vi "Insert_Event.vi"(0 "Alias Table":string[][](array[string])) -> (1 "Command":string, 2 "Cancelled":bool)   [LabVIEW 2011]
doc: "This modal VI functions as a popup window, allowing the user to select a new event to insert into the sequence."
panel:
  in  "Commands":i32(listbox)
  in  "Cancel":bool
  in  "OK":bool
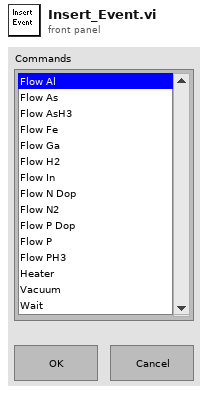
[diagram p1: front panel]
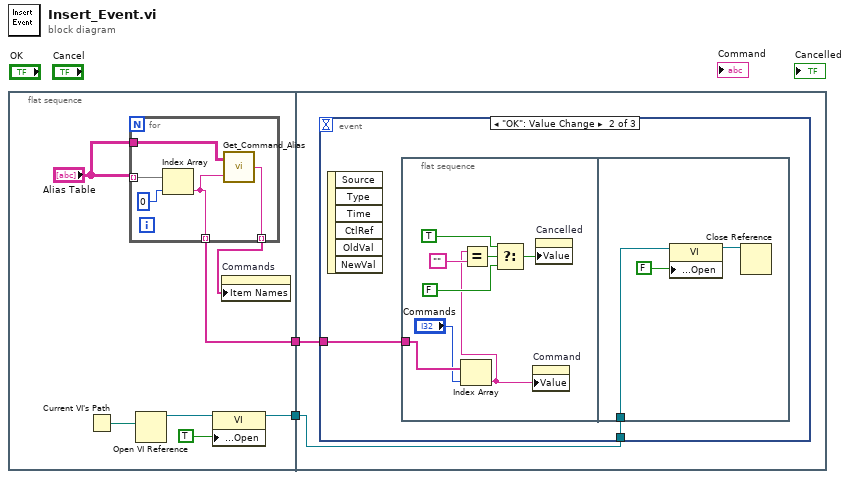
[diagram p0: block diagram]
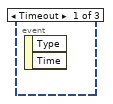
[diagram p2: hidden frame]
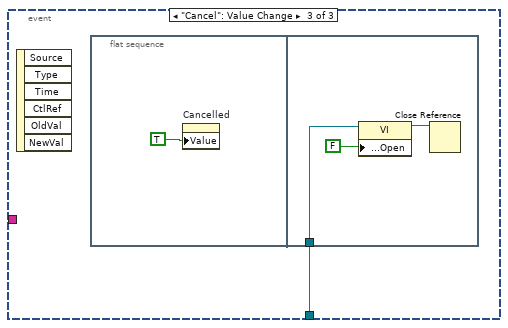
[diagram p3: hidden frame]
diagram:
  n1 = flat-sequence {
    tunnel: [w8] -> w2
    tunnel: [w4] -> w1
    tunnel: w2 -> [w16]
    tunnel: w1 -> [w15]
    frame #0 {
      n2 = Current VI's Path() -> (path=w6:path)
      n3 = for {
        tunnel: "Alias Table" -> [w13]
        tunnel: [w14] -> w5 mode=indexing
        tunnel: [w10] -> w4 mode=indexing
        tunnel: "Alias Table" -> [w12] mode=indexing
        n4 = Index Array(array=w12, index=0) -> (element=w10:string)
        n5 = call "Get_Command_Alias.vi"("Command"=w10, "Alias Table"=w13) -> ("Alias"=w14:string)
      }
      n6 = Open VI Reference(vi path=w6) -> (vi reference=w7:refnum<vi>)  [unwired: 1 in, 5 out]
      n7 = property class="VI"(reference=w7, "Front Panel.Open"=TRUE ("Front Panel Window:Open")) -> (reference out=w8:refnum<vi>)  [unwired: 1 in, 1 out]
      n8 = property on="Commands" class="LstBox (strict)"("Item Names"=w5) -> ()  [unwired: 2 in, 2 out]
    }
    frame #1 {
      n9 = event shown="[1] \"OK\": Value Change" {
        selector: _ -> [_ _ _]
        dyn-events: _ -> [_ _ _]
        timeout: _ -> [_ _ _]
        tunnel: w16 -> [_ w18 w30]
        tunnel: w15 -> [_ w17 _]
        event Timeout {
          n10 = event-data() -> ()  [unwired: 3 out]
        }
        event "OK": Value Change {
          n11 = event-data() -> ()  [unwired: 7 out]
          n12 = flat-sequence {
            tunnel: w17 -> [w21]
            tunnel: w18 -> [w28]
            frame #0 {
              n13 = Index Array(array=w21, index="Commands") -> (element=w19:string)
              n14 = Equal?(x=w19, y="") -> (x = y?=w23:bool)
              n15 = Select(t=TRUE ("Cancelled"), s=w23, f=FALSE) -> (s? t:f=w24:bool)
              n16 = property on="Command" class="Str"("Value"=w19) -> ()  [unwired: 2 in, 2 out]
              n17 = property on="Cancelled" class="Bool (strict)"("Value"=w24) -> ()  [unwired: 2 in, 2 out]
            }
            frame #1 {
              n18 = property class="VI"(reference=w28, "Front Panel.Open"=FALSE ("Front Panel Window:Open")) -> (reference out=w27:refnum<vi>)  [unwired: 1 in, 1 out]
              n19 = Close Reference(reference=w27) -> ()  [unwired: 1 in, 1 out]
            }
          }
        }
        event "Cancel": Value Change {
          n20 = event-data() -> ()  [unwired: 7 out]
          n21 = flat-sequence {
            tunnel: w30 -> [w33]
            frame #0 {
              n22 = property on="Cancelled" class="Bool (strict)"("Value"=TRUE ("Cancelled")) -> ()  [unwired: 2 in, 2 out]
            }
            frame #1 {
              n23 = property class="VI"(reference=w33, "Front Panel.Open"=FALSE ("Front Panel Window:Open")) -> (reference out=w32:refnum<vi>)  [unwired: 1 in, 1 out]
              n24 = Close Reference(reference=w32) -> ()  [unwired: 1 in, 1 out]
            }
          }
        }
      }
    }
  }
